vi "Get Gif Logical Screen Descriptor.vi"(8 "error in (no error)":errorcluster caption="错误输入（无错误）", 11 "Gif Image 输入":refnum<class "Gif Image.lvclass"> caption="DNL_LabVIEW Object in") -> (0 "error out":errorcluster caption="错误输出", 3 "Gif Image 输出":refnum<class "Gif Image.lvclass"> caption="DNL_LabVIEW Object out")   [LabVIEW 2012, in "Picture Box Tools.lvlib" / "Gif Image.lvclass"]
uses:
  Gif Image.lvclass
  Control/Logical Screen Descriptor.ctl
  Gif Image.lvclass/Gif Image.ctl
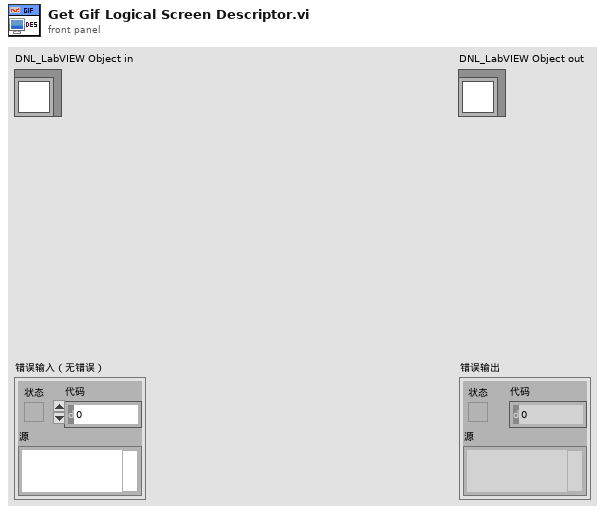
[diagram p1: front panel]
types:
  T1 = enum16{"big-endian, network order", "native, host order", "little-endian"}
  T2 = typedef "Picture Box Tools.lvlib/Gif Image.lvclass/Logical Screen Descriptor.ctl" = cluster{"Logical Screen Width":u16, "Logical Screen Height":u16, "Pack Field":u8, "Background Color Index":u8, "Pixel Aspect Ratio":u8}
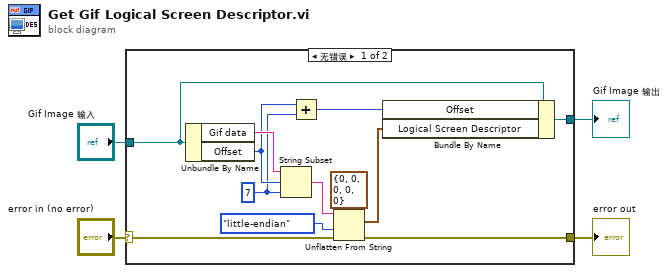
[diagram p0: block diagram]
diagram:
  n1 = case shown="无错误" "error in (no error)" {
    selector: "error in (no error)" -> [w12 w18]
    tunnel: [w11 w18] -> w3
    tunnel: [w9 w17] -> w1
    tunnel: "Gif Image 输入" -> [w10 w17]
    frame No Error {
      w7 = 7 ("长度（剩余）")
      n2 = Unbundle By Name(w10) -> ("Gif data"=w16:string, "Offset"=w8:i32)
      n3 = String Subset(string=w16, offset (0)=w8, length (rest)=w7) -> (substring=w15:string)
      n4 = Add(x=w8, y=w7) -> (x+y=w6:i32)
      n5 = Unflatten From String(type=T2 {"Logical Screen Width"=0, "Logical Screen Height"=0, "Pack Field"=0, "Background Color Index"=0, "Pixel Aspect Ratio"=0} ("Logical Screen Descriptor Out"), binary string=w15, byte order (0:big-endian, network order)=T1."little-endian" ("字节顺序(0:big-endian, network order)"), error in (no error)=w12) -> (value=w5:T2, error out=w11:errorcluster)  [unwired: 1 in, 1 out]
      n6 = Bundle By Name(cluster=w10, "Offset"=w6, "Logical Screen Descriptor"=w5) -> (w9:refnum<class "Gif Image.lvclass">)
    }
    frame Error {
    }
  }
  "error out" <- w3
  "Gif Image 输出" <- w1
